vi "multi_port.vi"() -> ()   [LabVIEW 2016]
uses:
  dxl_x86_c.lvlib/dxl_x86_c.lvlib
panel:
  out "value : PRO (knob)\npresent position 2":i32(knob) scale=150000.0..-150000.0
  in  "device_name2":string="COM2"
  out "port_num2":i32
  in  "dynamixe2_id":u8=2
  in  "device_name1":string="COM1"
  in  "ADDR_PRO_\nPRESENT_POSITION":u16=611
  in  "ADDR_PRO_\nGOAL_POSITION":u16=596
  in  "ADDR_PRO_\nTORQUE_ENABLE":u16=562
  out "protocol_version":dbl=2.0
  out "value : PRO (knob)\npresent position 1":i32(knob) scale=150000.0..-150000.0
  in  "terminate":bool
  out "port_num1":i32
  in  "value : PRO (dial)\ngoal position":i32(knob) scale=150000.0..-150000.0
  in  "dynamixel1_id":u8=1
  in  "baud_rate":i32=1000000
  # "/*******************************************************************************\n* Copyright (c) 2016, ROBOTIS CO., LTD.\n* All rights reserved.\n*\n* Redistribution and use in source and binary forms, with or without\n* modification, are permitted provided that the following conditions are met:\n*\n* * Redistributions of source code must retain the above copyright notice, this\n*   list of conditions and the following disclaimer.\n*\n* * Redistributions in binary form must reproduce the above copyright notice,\n*   this list of conditions and the following disclaimer in the documentation\n*   and/or other materials provided with the distribution.\n*\n* * Neither the name of ROBOTIS nor the names of its\n*   contributors may be used to endorse or promote products derived from\n*   this software without specific prior written permission.\n*\n* THIS SOFTWARE IS PROVIDED BY THE COPYRIGHT HOLDERS AND CONTRIBUTORS \"AS IS\"\n* AND ANY EXPRESS OR IMPLIED WARRANTIES, INCLUDING, BUT NOT LIMITED TO, THE\n* IMPLIED WARRANTIES OF MERCHANTABILITY AND FITNESS FOR A PARTICULAR PURPOSE ARE\n* DISCLAIMED. IN NO EVENT SHALL THE COPYRIGHT HOLDER OR CONTRIBUTORS BE LIABLE\n* FOR ANY DIRECT, INDIRECT, INCIDENTAL, SPECIAL, EXEMPLARY, OR CONSEQUENTIAL\n* DAMAGES (INCLUDING, BUT NOT LIMITED TO, PROCUREMENT OF SUBSTITUTE GOODS OR\n* SERVICES; LOSS OF USE, DATA, OR PROFITS; OR BUSINESS INTERRUPTION) HOWEVER\n* CAUSED AND ON ANY THEORY OF LIABILITY, WHETHER IN CONTRACT, STRICT LIABILITY,\n* OR TORT (INCLUDING NEGLIGENCE OR OTHERWISE) ARISING IN ANY WAY OUT OF THE USE\n* OF THIS SOFTWARE, EVEN IF ADVISED OF THE POSSIBILITY OF SUCH DAMAGE.\n*******************************************************************************/\n\n/* Author: Ryu Woon Jung (Leon) */"
  # "Available Dynamixel model on this example : All models using Protocol 2.0\nThis example is designed for using two Dynamixel PRO 54-200, and two USB2DYNAMIXEL.\nTo use another Dynamixel model, such as X series, see their details in E-Manual(support.robotis.com) \n   and edit \"numeric control\"s seen left with \"Edit Text\" tool.\nBe sure that Dynamixel PRO properties are already set as %% ID : 1 / Baudnum : 1 (Baudrate : 57600)\n\n\n1. Run example by click above \"Run\" button (below \"Edit\" menu).\n2. Drag \"dial\" then you may see the Dynamixel and \"knob\"s rotating\n3. To finish the example, press \"terminate\" button."
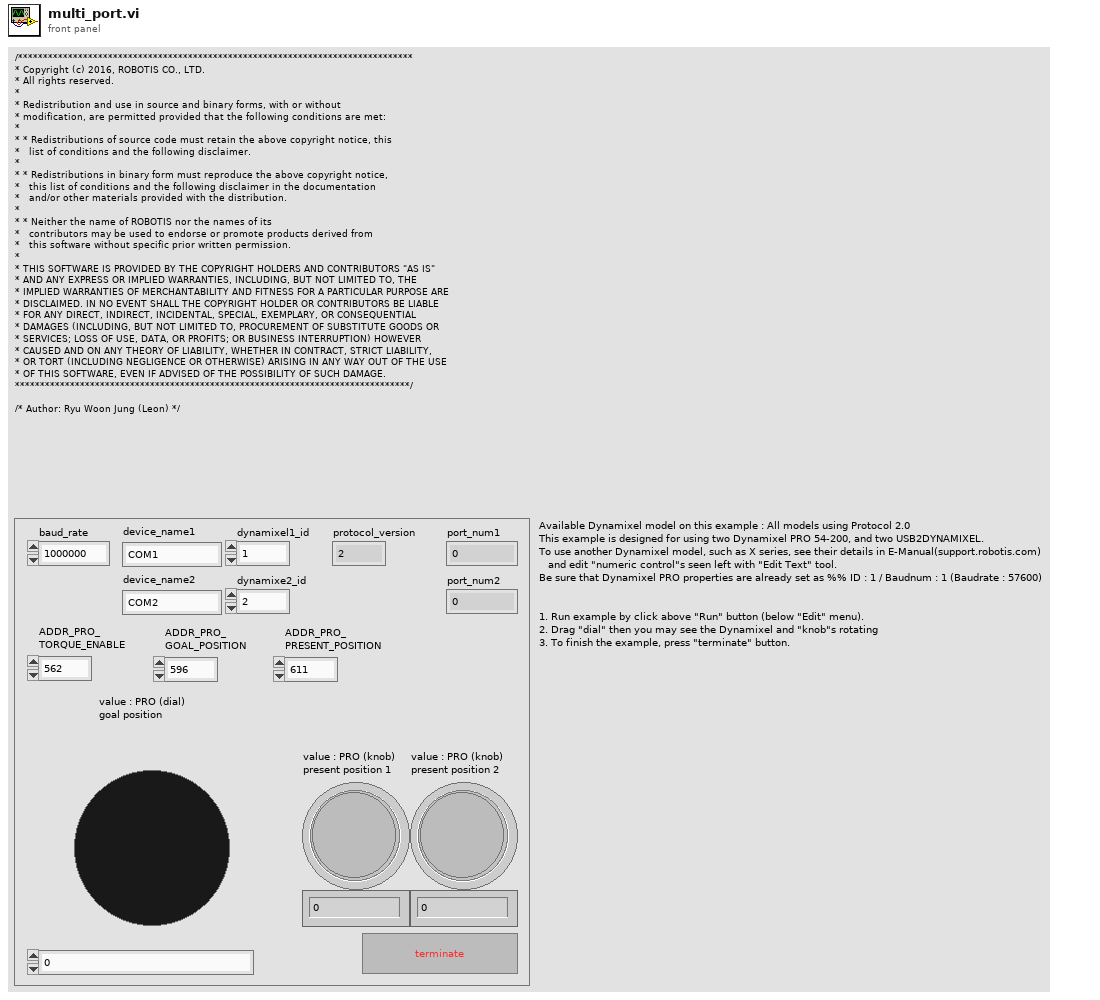
[diagram p1: front panel]
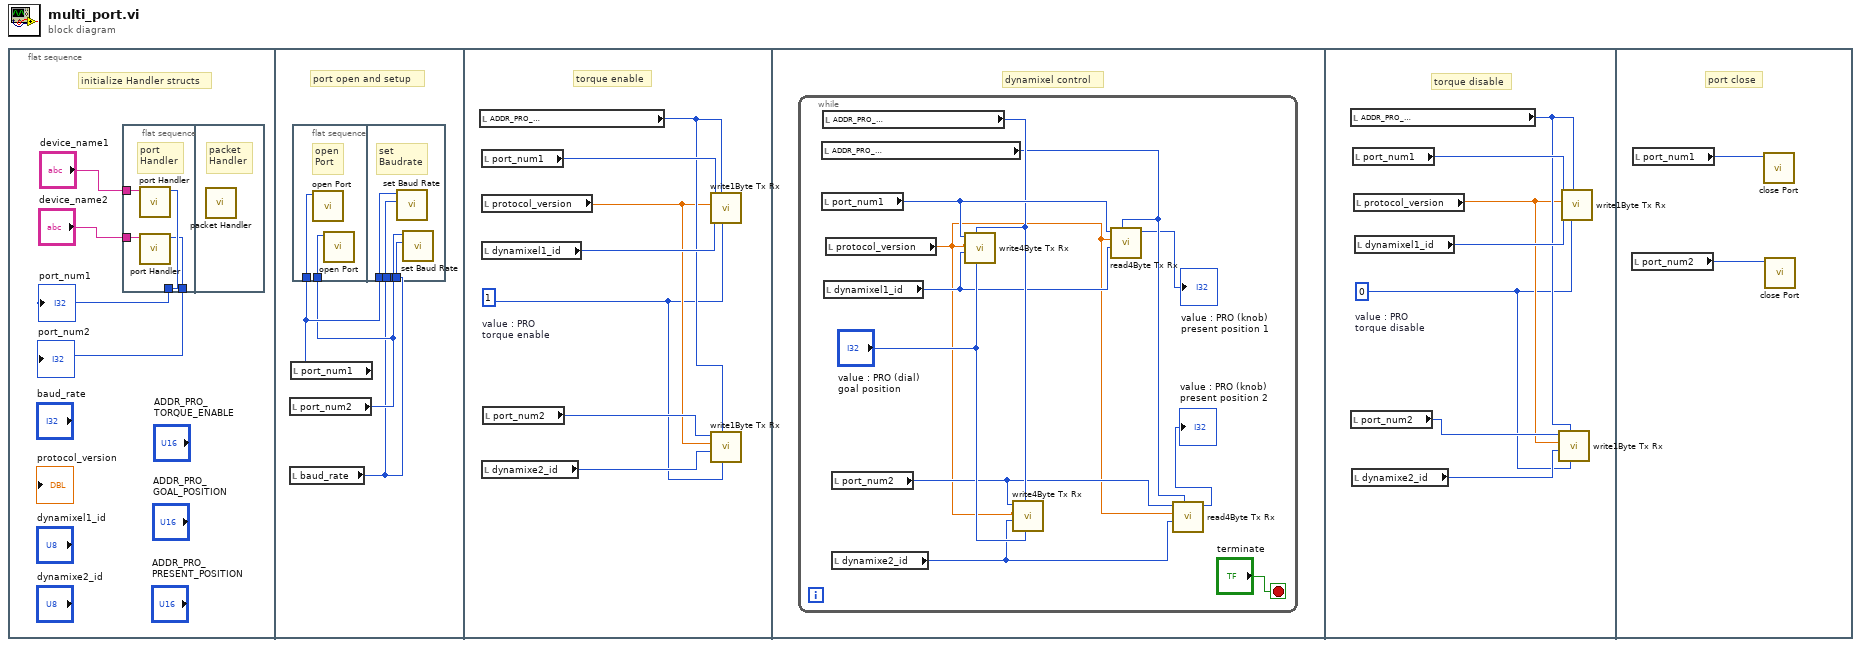
[diagram p0: block diagram]
diagram:
  n1 = flat-sequence {
    frame #0 {
      # "initialize Handler structs"
      n2 = flat-sequence {
        tunnel: "device_name1" -> [w8]
        tunnel: "device_name2" -> [w7]
        tunnel: [w6] -> w2
        tunnel: [w5] -> w1
        frame #0 {
          # "port\nHandler"
          n3 = call "port Handler.vi"("port_name"=w8) -> ("function return"=w6:i32)  [unwired: 10 in]
          n4 = call "port Handler.vi"("port_name"=w7) -> ("function return"=w5:i32)  [unwired: 10 in]
        }
        frame #1 {
          # "packet\nHandler"
          n5 = call "packet Handler.vi"() -> ()  [unwired: 12 in]
        }
      }
      "port_num1" <- w2
      "port_num2" <- w1
    }
    frame #1 {
      # "port open and setup"
      n6 = local read "port_num2"() -> (w10:i32)
      n7 = local read "baud_rate"() -> (w9:i32)
      n8 = local read "port_num1"() -> (w11:i32)
      n9 = flat-sequence {
        tunnel: w11 -> [w13]
        tunnel: w10 -> [w12]
        tunnel: w11 -> [w17]
        tunnel: w9 -> [w16]
        tunnel: w10 -> [w15]
        tunnel: w9 -> [w14]
        frame #0 {
          # "open\nPort"
          n10 = call "open Port.vi"("port_num"=w13) -> ()  [unwired: 10 in, 1 out]
          n11 = call "open Port.vi"("port_num"=w12) -> ()  [unwired: 10 in, 1 out]
        }
        frame #1 {
          # "set\nBaudrate"
          n12 = call "set Baud Rate.vi"("baudrate"=w16, "port_num"=w17) -> ()  [unwired: 9 in, 1 out]
          n13 = call "set Baud Rate.vi"("baudrate"=w14, "port_num"=w15) -> ()  [unwired: 9 in, 1 out]
        }
      }
    }
    frame #2 {
      w18 = 1  # value : PRO torque enable
      # "torque enable"
      n14 = local read "ADDR_PRO_\nTORQUE_ENABLE"() -> (w22:u16)
      n15 = local read "port_num1"() -> (w23:i32)
      n16 = local read "protocol_version"() -> (w20:dbl)
      n17 = local read "dynamixel1_id"() -> (w24:u8)
      n18 = local read "dynamixe2_id"() -> (w19:u8)
      n19 = local read "port_num2"() -> (w21:i32)
      n20 = call "write1Byte Tx Rx.vi"("data"=w18, "address"=w22, "id"=w24, "protocol_version"=w20, "port_num"=w23) -> ()  [unwired: 7 in]
      n21 = call "write1Byte Tx Rx.vi"("data"=w18, "address"=w22, "id"=w19, "protocol_version"=w20, "port_num"=w21) -> ()  [unwired: 7 in]
    }
    frame #3 {
      # "dynamixel control"
      n22 = while {
        stop <- "terminate" stop-if-true
        n23 = local read "ADDR_PRO_\nPRESENT_POSITION"() -> (w30:u16)
        n24 = local read "port_num1"() -> (w34:i32)
        n25 = local read "ADDR_PRO_\nGOAL_POSITION"() -> (w32:u16)
        n26 = local read "dynamixel1_id"() -> (w31:u8)
        n27 = local read "protocol_version"() -> (w25:dbl)
        n28 = local read "port_num2"() -> (w26:i32)
        n29 = local read "dynamixe2_id"() -> (w27:u8)
        n30 = call "write4Byte Tx Rx.vi"("data"="value : PRO (dial)\ngoal position", "address"=w32, "id"=w31, "protocol_version"=w25, "port_num"=w34) -> ()  [unwired: 7 in]
        n31 = call "write4Byte Tx Rx.vi"("data"="value : PRO (dial)\ngoal position", "address"=w32, "id"=w27, "protocol_version"=w25, "port_num"=w26) -> ()  [unwired: 7 in]
        n32 = call "read4Byte Tx Rx.vi"("address"=w30, "id"=w31, "protocol_version"=w25, "port_num"=w34) -> ("function return"=→"value : PRO (knob)\npresent position 1":u32)  [unwired: 7 in]
        n33 = call "read4Byte Tx Rx.vi"("address"=w30, "id"=w27, "protocol_version"=w25, "port_num"=w26) -> ("function return"=→"value : PRO (knob)\npresent position 2":u32)  [unwired: 7 in]
      }
    }
    frame #4 {
      w36 = 0  # value : PRO torque disable
      # "torque disable"
      n34 = local read "ADDR_PRO_\nTORQUE_ENABLE"() -> (w40:u16)
      n35 = local read "port_num2"() -> (w39:i32)
      n36 = local read "dynamixe2_id"() -> (w37:u8)
      n37 = local read "port_num1"() -> (w42:i32)
      n38 = local read "protocol_version"() -> (w38:dbl)
      n39 = local read "dynamixel1_id"() -> (w41:u8)
      n40 = call "write1Byte Tx Rx.vi"("data"=w36, "address"=w40, "id"=w37, "protocol_version"=w38, "port_num"=w39) -> ()  [unwired: 7 in]
      n41 = call "write1Byte Tx Rx.vi"("data"=w36, "address"=w40, "id"=w41, "protocol_version"=w38, "port_num"=w42) -> ()  [unwired: 7 in]
    }
    frame #5 {
      # "port close"
      n42 = local read "port_num2"() -> (w43:i32)
      n43 = local read "port_num1"() -> (w44:i32)
      n44 = call "close Port.vi"("port_num"=w44) -> ()  [unwired: 11 in]
      n45 = call "close Port.vi"("port_num"=w43) -> ()  [unwired: 11 in]
    }
  }
